vi "DSF.Engine.Framework.Set Transceiver Loader.vi"(10 "Transceiver Loader":refnum<class "Transceiver Loader.lvclass">, 11 "Framework in":refnum<class "DSF.Engine.Framework.lvclass">) -> (3 "Framework out":refnum<class "DSF.Engine.Framework.lvclass">)   [LabVIEW 2017, in "Data Sharing Framework Engine.lvlib" / "DSF.Engine.Framework.lvclass"]
uses:
  DSF.Engine.Framework.lvclass
  Source/Data Sharing Framework Core/Engine/Transceiver/Transceiver Loader/Transceiver Loader.lvclass
  DSF.Engine.Framework.lvclass/DSF.Engine.Framework.ctl
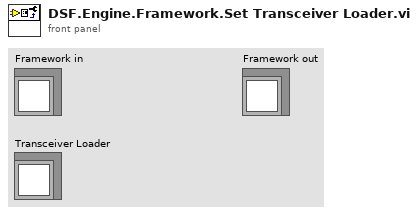
[diagram p1: front panel]
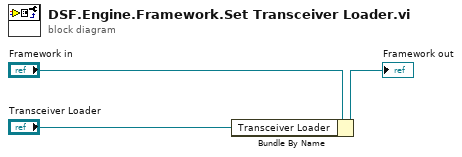
[diagram p0: block diagram]
diagram:
  n1 = Bundle By Name(cluster="Framework in", "Transceiver Loader"="Transceiver Loader") -> (→"Framework out":refnum<class "DSF.Engine.Framework.lvclass">)
